vi "foucault display panel.vi"() -> ()   [LabVIEW 2017]
uses:
  <vilib>/Instr/_visa.llb/VISA Set IO Buffer Mask.ctl
  <vilib>/Platform/TimedLoop/XDataNode/timing_clust.ctl
  <vilib>/Platform/TimedLoop/XDataNode/nitl_modes.ctl
  <vilib>/Platform/TimedLoop/XDataNode/wakeup.ctl
  <vilib>/Instr/_visa.llb/VISA Configure Serial Port (Instr).vi
  <vilib>/platform/TimedLoop/XDataNode/XDataNode.xnode
  <vilib>/Platform/TimedLoop/XDataNode/XDNodeRunTimeDep.lvlib
panel:
  out "size(s)":i32
  out "min index(es)":i32
  out "min value":dbl
  out "max index(es)":i32
  out "max value":dbl
  in  "stop":bool
  in  "graphy type":enum16{"voltage and coil", "mag x and y"}(ring)
  in  "slope":bool
  in  "hysteresis (mV)":dbl format="%#_6f"
  in  "trigger?":bool
  in  "relative to crossing":dbl
  in  "sample length":i32=5000
  out "z accel":dbl format="%0.2f"
  out "Yaccel":dbl(slide) scale=-1.0..1.0
  out "Xaccel":dbl(slide) scale=-1.0..1.0
  in  "reset":bool
  out "deg/hr":dbl format="%0.2f"
  out "angle vs time":cluster{dbl[], dbl[]}[](graph)
  out "angle":dbl
  out "mag slope":dbl
  out "magnet":cluster{dbl[], dbl[]}[](graph)
  in  "sliding window":dbl=2.2 format="%#_13g"
  in  "stop 2":bool
  out "voltage":cluster{dbl[], dbl[]}[](graph)
  in  "update (ms)":i64=100
  out "error out":errorcluster
  in  "VISA resource name":refnum<visa-resource-name>
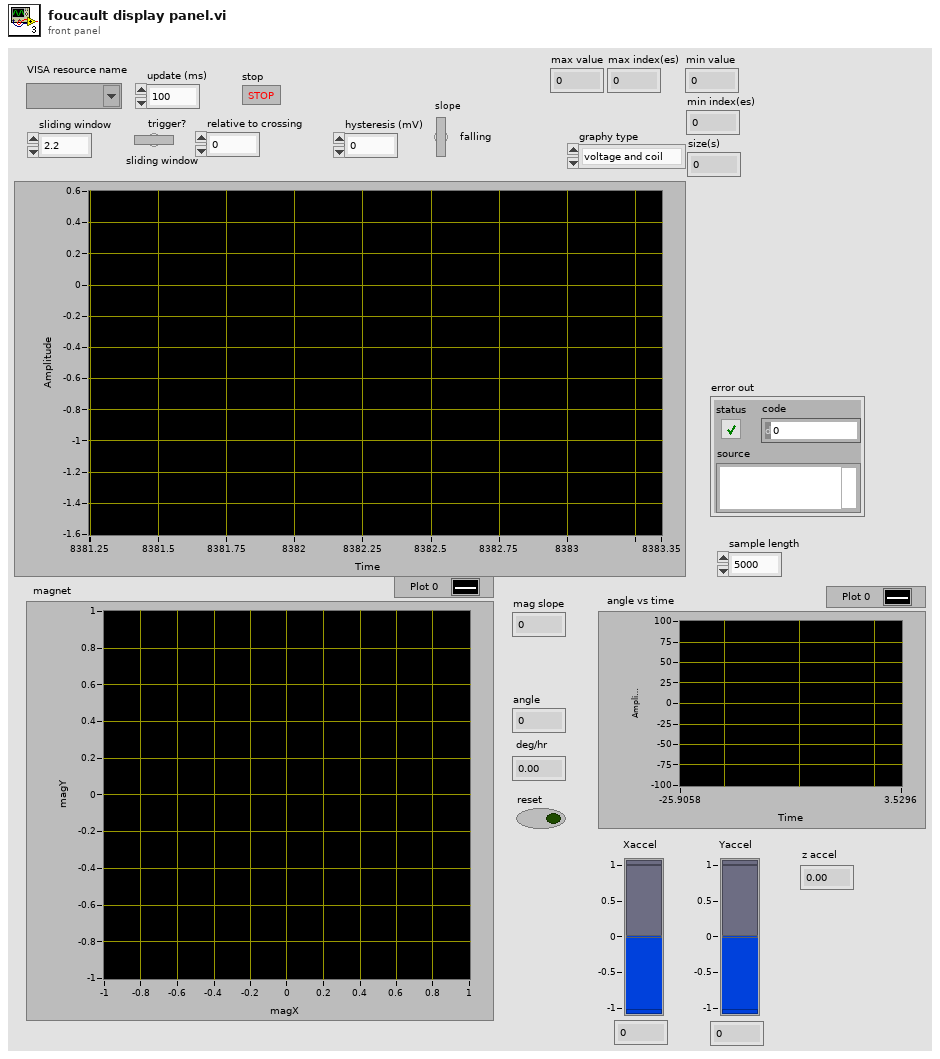
[diagram p1: front panel]
types:
  T1 = typedef "VISA Set IO Buffer Mask.ctl" = u16
  T2 = cluster{"voltage":refnum<queue>, "coil":refnum<queue>, "mag":refnum<queue>, "accel":refnum<queue>}
  T3 = typedef "XDNodeRunTimeDep.lvlib/timing_clust.ctl" = cluster{"Expected End [f-1]":u64, "Actual End [f-1]":u64, "Finished Late? [f-1]":bool, "Expected End [i-1]":u64, "Actual End [i-1]":u64, "Finished Late? [i-1]":bool, "Expected Start [i]":u64, "Actual Start [i]":u64, "Expected Start [f]":u64, "Actual Start [f]":u64, "Source Name":string, "Structure Name":string, "Period":i64, "Deadline":i64, "Offset":i64, "Start":i64, "Priority":i32, "Timeout":i32, "Mode":T4, "Wakeup Reason":T5, "Error":errorcluster, "Source Type":string, "Secondary Source Type":string, "Global End Time":u64, "Global Start Time":u64, "Frame Duration":u64, "Iteration Duration":u64, "Assigned CPU":i32, "I/O Scan Engine Mode":u32}
  T4 = typedef "XDNodeRunTimeDep.lvlib/nitl_modes.ctl" = enum32{"No Change", "Process missed periods, maintain original phase", "Discard missed periods, maintain original phase", "Process missed periods, ignore original phase", "Discard missed periods, ignore original phase"}
  T5 = typedef "XDNodeRunTimeDep.lvlib/wakeup.ctl" = enum32{"Normal", "Aborted", "Asynchronous wakeup", "Timing source error", "Timed loop error", "Timeout"}
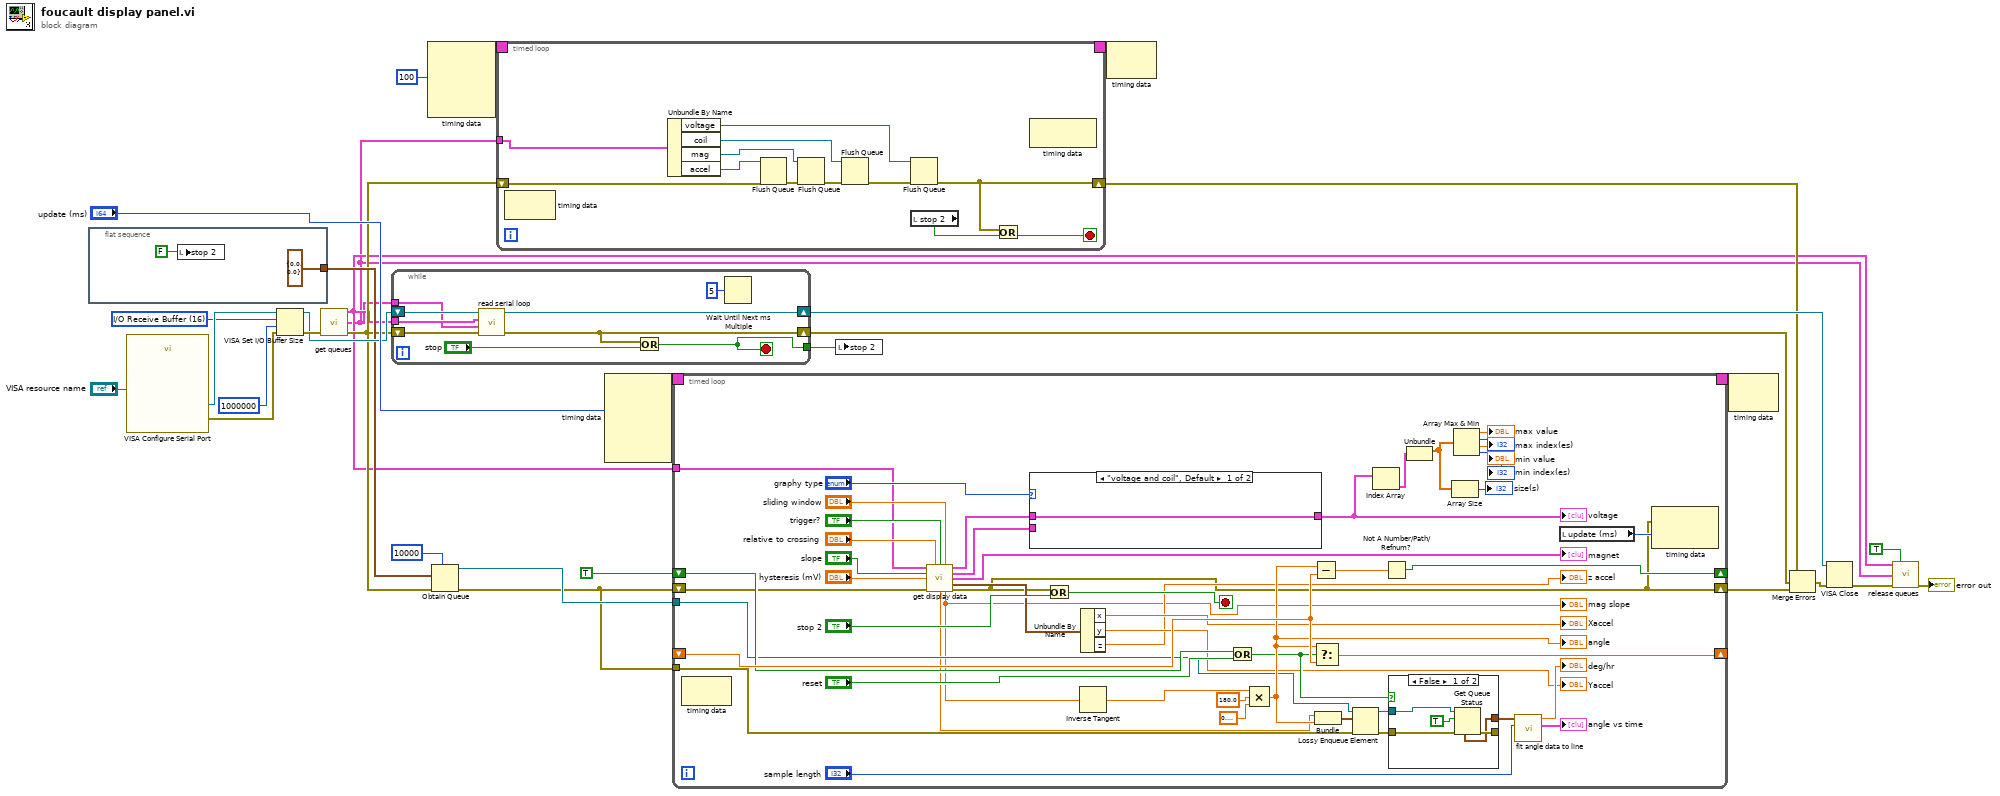
[diagram p0: block diagram]
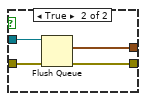
[diagram p3: hidden frame]
diagram:
  w27 = T1 16 items=["I/O Receive Buffer"=16, "I/O Transmit Buffer"=32, "I/O Receive and Transmit Buffer"=48] ("Mask")
  n1 = flat-sequence {
    tunnel: [cluster{"mean":dbl, dbl} {"mean"=0.0, 0.0} ("output cluster")] -> w16
    frame #0 {
      n2 = local write "stop 2"(FALSE ("stop 2")) -> ()
    }
  }
  n3 = call-poly "VISA Configure Serial Port"("VISA resource name"="VISA resource name") -> ("VISA resource name out"=w29:refnum<visa-resource-name>, "error out"=w26:errorcluster)  [unwired: 13 in]
  n4 = VISA Set I/O Buffer Size(VISA resource name=w29, mask (16)=w27, size (4096)=u32 1000000, error in (no error)=w26) -> (VISA resource name out=w18:refnum<visa-resource-name>, error out=w19:errorcluster)
  n5 = call "get queues.vi"("error in (no error)"=w19) -> ("display queues"=w2:T2, "disk queues"=w1:T2, "error out"=w4:errorcluster)  [unwired: 12 in]
  n6 = while {
    tunnel: [w37] -> w15
    shift-right: [w38] -> w11
    shift-left: w18 -> [w40]
    shift-right: [w36] -> w12
    shift-left: w4 -> [w41]
    tunnel: w2 -> [w34]
    tunnel: w1 -> [w33]
    stop <- w37 stop-if-true
    n7 = call "read serial loop.vi"("error in (no error)"=w41, "disk queues"=w33, "display queues"=w34, "serial port"=w40) -> ("error out"=w36:errorcluster, "VISA resource name out"=w38:refnum<visa-resource-name>)  [unwired: 6 in]
    n8 = Or(x=w36, y="stop") -> (x .or. y?=w37:bool)
    n9 = Wait Until Next ms Multiple(millisecond multiple=u32 5) -> ()  [unwired: 1 out]
  }
  n10 = node-c288(i64 100 ("Period")) -> (w7:T3)  [unwired: 3 in]
  n11 = Obtain Queue(max queue size (-1, unlimited)=10000, element data type=w16, error in (no error)=w4) -> (queue out=w21:refnum<queue>, error out=w17:errorcluster)  [unwired: 2 in, 1 out]
  n12 = timed-loop {
    timing: w7 -> [_]
    timing-out: [_] -> w6
    shift-right: [w45] -> w3
    shift-left: w4 -> [w53]
    tunnel: w1 -> [w42]
    stop <- w44 stop-if-true
    n13 = node-c288() -> ()  [unwired: 1 in, 1 out]
    n14 = Unbundle By Name(w42) -> ("voltage"=w43:refnum<queue>, "coil"=w51:refnum<queue>, "mag"=w50:refnum<queue>, "accel"=w49:refnum<queue>)
    n15 = Flush Queue(queue=w49, error in (no error)=w53) -> (error out=w48:errorcluster)  [unwired: 2 out]
    n16 = Flush Queue(queue=w50, error in (no error)=w48) -> (error out=w47:errorcluster)  [unwired: 2 out]
    n17 = Flush Queue(queue=w51, error in (no error)=w47) -> (error out=w46:errorcluster)  [unwired: 2 out]
    n18 = Flush Queue(queue=w43, error in (no error)=w46) -> (error out=w45:errorcluster)  [unwired: 2 out]
    n19 = local read "stop 2"() -> (w52:bool)
    n20 = Or(x=w45, y=w52) -> (x .or. y?=w44:bool)
    n21 = node-c288() -> ()  [unwired: 1 in, 1 out]
  }
  n22 = node-c288("update (ms)") -> (w25:T3)  [unwired: 4 in]
  n23 = timed-loop {
    timing: w25 -> [_]
    timing-out: [_] -> w24
    shift-right: [w99] -> _
    shift-left: _ -> [w98]
    shift-right: [w97] -> _
    shift-left: TRUE -> [w96]
    shift-right: [w67] -> w14
    shift-left: w17 -> [w74]
    tunnel: w21 -> [w91]
    tunnel: w17 -> [w89]
    tunnel: w2 -> [w56]
    stop <- w93 stop-if-true
    n24 = node-c288() -> ()  [unwired: 1 in, 1 out]
    n25 = call "get display data.vi"("display queues"=w56, "relative to crossing"="relative to crossing", "trigger?"="trigger?", "sliding window"="sliding window", "slope"="slope", "hysteresis (mV)"="hysteresis (mV)", "error in (no error)"=w74) -> ("voltage vs t"=w76:cluster{dbl[], dbl[]}[], "mag vs t"=w75:cluster{dbl[], dbl[]}[], "mag xy last cycle"=→"magnet":cluster{dbl[], dbl[]}[], "accelerometer reading"=w73:cluster{"x":dbl, "y":dbl, "z":dbl}, "mag slope time"=w68:dbl, "mag slope"=w69:dbl, "error out"=w67:errorcluster)  [unwired: 2 in]
    "mag slope" <- w69
    n26 = case shown="\"voltage and coil\", Default" "graphy type" {
      tunnel: w76 -> [w105 _]
      tunnel: w75 -> [_ w106]
      tunnel: [w105 w106] -> w66
      frame "voltage and coil", Default {
      }
      frame "mag x and y" {
      }
    }
    "voltage" <- w66
    n27 = Or(x=w67, y="stop 2") -> (x .or. y?=w93:bool)
    n28 = Inverse Tangent(1:w69) -> (0:w102:dbl)
    n29 = Unbundle By Name(w73) -> ("x"=→"Xaccel":dbl, "y"=→"Yaccel":dbl, "z"=→"z accel":dbl)
    n30 = Or(x=w96, y="reset") -> (x .or. y?=w88:bool)
    n31 = Compound Arithmetic op=MULTIPLY(w102, 180.0 ("y"), 0.3183098861837907) -> (w92:dbl)
    "angle" <- w92
    n32 = Subtract(x=w92, y=w98) -> (x-y=w95:dbl)
    n33 = Select(t=w92, s=w88, f=w98) -> (s? t:f=w99:dbl)
    n34 = Bundle("mag slope time"=w68, w92) -> (w90:cluster{"mag slope time":dbl, dbl})  [unwired: 1 in]
    n35 = Lossy Enqueue Element(queue=w91, element=w90, error in (no error)=w89) -> (queue out=w87:refnum<queue>, error out=w86:errorcluster)  [unwired: 2 out]
    n36 = Index Array(array=w66) -> (element=w65:cluster{dbl[], dbl[]})  [unwired: 1 in]
    n37 = Not A Number/Path/Refnum?(number/path/refnum=w95) -> (NaN/Path/Refnum?=w97:bool)
    n38 = case shown="False" w88 {
      tunnel: w87 -> [w111 w115]
      tunnel: w86 -> [w109 w114]
      tunnel: [w107 w113] -> w85
      tunnel: [w108 w112] -> _
      frame False {
        n39 = Get Queue Status(queue=w111, return elements? (F)=TRUE, error in (no error)=w109) -> (error out=w108:errorcluster, elements=w107:cluster{"mean":dbl, dbl}[])  [unwired: 6 out]
      }
      frame True {
        n40 = Flush Queue(queue=w115, error in (no error)=w114) -> (remaining elements=w113:cluster{"mean":dbl, dbl}[], error out=w112:errorcluster)  [unwired: 1 out]
      }
    }
    n41 = Unbundle(w65) -> (w60:dbl[])  [unwired: 1 out]
    n42 = Array Size(array=w60) -> (size(s)=→"size(s)":i32)
    n43 = Array Max & Min(array=w60) -> (max value=→"max value":dbl, max index (indices)=→"max index(es)":i32, min value=→"min value":dbl, min index (indices)=→"min index(es)":i32)
    n44 = call "fit angle data to line.vi"("length"="sample length", "remaining elements"=w85) -> ("graphs"=→"angle vs time":cluster{dbl[], dbl[]}[], "deg/hr"=→"deg/hr":dbl)  [unwired: 8 in]
    n45 = local read "update (ms)"() -> (w104:i64)
    n46 = node-c288(w67, w104) -> ()  [unwired: 1 out]
  }
  n47 = local write "stop 2"(w15) -> ()
  n48 = node-c288(w6) -> ()  [unwired: 1 out]
  n49 = node-c288(w24) -> ()  [unwired: 1 out]
  n50 = Merge Errors(w3, w12, w14) -> (w13:errorcluster)
  n51 = VISA Close(VISA resource name=w11, error in (no error)=w13) -> (error out=w10:errorcluster)
  n52 = call "release queues.vi"("display queues"=w2, "force destroy? (F)"=TRUE, "disk queues"=w1, "error in (no error)"=w10) -> ("error out"=→"error out":errorcluster)  [unwired: 11 in]
